vi "Wait on Transport Notification.vi"(8 "error in (no error)":errorcluster, 9 "Timeout In ms (-1)":i32=-1, 10 "ignore previous (F)":bool, 11 "NotifierTransport":refnum<class "NotifierTransport.lvclass">) -> (0 "error out":errorcluster, 1 "Publication Time":timestamp, 2 "Data":variant)   [LabVIEW 2017, in "NotifierTransport.lvclass"]
uses:
  NotifierTransport.lvclass
  NotifierTransport.lvclass/NotifierTransport.ctl
  <vilib>/Utility/error.llb/Error Cluster From Error Code.vi
  <vilib>/ErrorRing/Error Ring.xnode
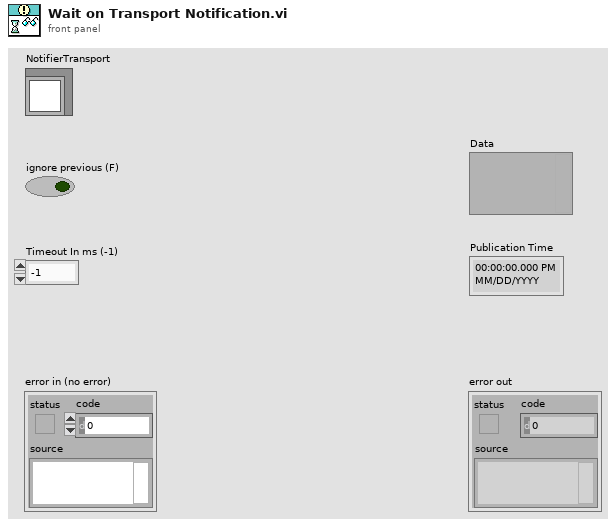
[diagram p1: front panel]
types:
  T1 = cluster{"Data":variant, "Publication Time":timestamp}
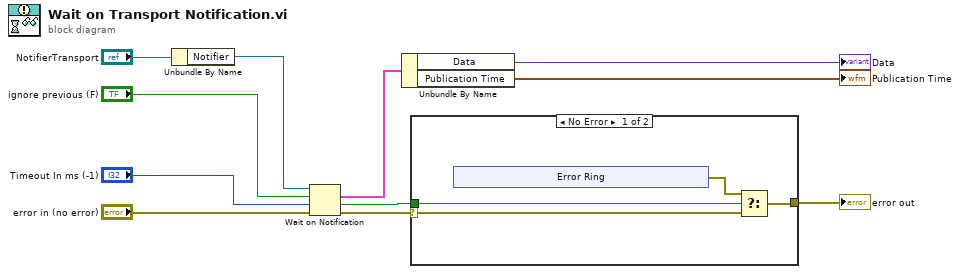
[diagram p0: block diagram]
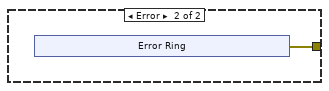
[diagram p2: hidden frame]
diagram:
  n1 = Unbundle By Name("NotifierTransport") -> ("Notifier"=w5:refnum<notifier>)
  n2 = Wait on Notification(notifier=w5, ignore previous (F)="ignore previous (F)", timeout in ms (-1)="Timeout In ms (-1)", error in (no error)="error in (no error)") -> (notification=w8:T1, timed out?=w2:bool, error out=w3:errorcluster)  [unwired: 1 out]
  n3 = Unbundle By Name(w8) -> ("Data"=→"Data":variant, "Publication Time"=→"Publication Time":timestamp)
  n4 = case shown="No Error" w3 {
    selector: w3 -> [w13 _]
    tunnel: [w15 w21] -> w1
    tunnel: w2 -> [w14 _]
    frame No Error {
      n5 = xnode "Error Ring"() -> ("error out"=w12:errorcluster)
      n6 = Select(t=w12, s=w14, f=w13) -> (s? t:f=w15:errorcluster)
    }
    frame Error {
      n7 = xnode "Error Ring"() -> ("error out"=w21:errorcluster)
    }
  }
  "error out" <- w1
